vi "AVI Codec Comparison.vi"() -> ()   [LabVIEW 2014]
doc: "This example creates a new AVI for each compression filter installed on your computer and compares the size of the AVI file, the average write time, and the quality of the compressed AVI.\n\nThis example might take a few seconds to create all the AVIs required for analysis. The VI saves the AVIs in the temporary directory, which you set by selecting Tools>>Options, then selecting Paths from the top drop-down listbox."
uses:
  <vilib>/Analysis/baseanly.llb/Mean (DBL).vi
  <vilib>/vision/NI_Vision_Development_Module.lvlib
  <vilib>/Analysis/NI_AALBase.lvlib
panel:
  out "Results":i32(listbox)=-1
  out "Progress Bar":i32(slide) max=11 scale=0.0..11.0
  # "Overview: Demonstrates how to use the IMAQ AVI functions to compare the available codecs on the system and evaluate the codecs based on the resulting AVI size, write speed, and quality.\nRequirements: Vision Development Software.\nInstructions: Run the VI."
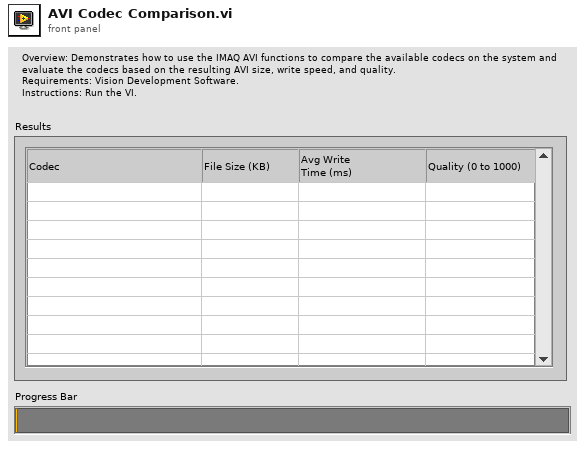
[diagram p1: front panel]
types:
  T1 = typedef "Image Type" = u32
  T2 = typedef "IMAQ Image.ctl" = refnum<image>
  T3 = typedef "IMAQ AVI2 Refnum.ctl" = refnum<k20>
  T4 = cluster{"histogram":u32[], "Minimal Value":sgl, "Maximal Value":sgl, "Starting Value":sgl, "Interval Width":sgl, "Mean Value":sgl, "Standard  Variation":sgl, "Area (pixels)":i32}
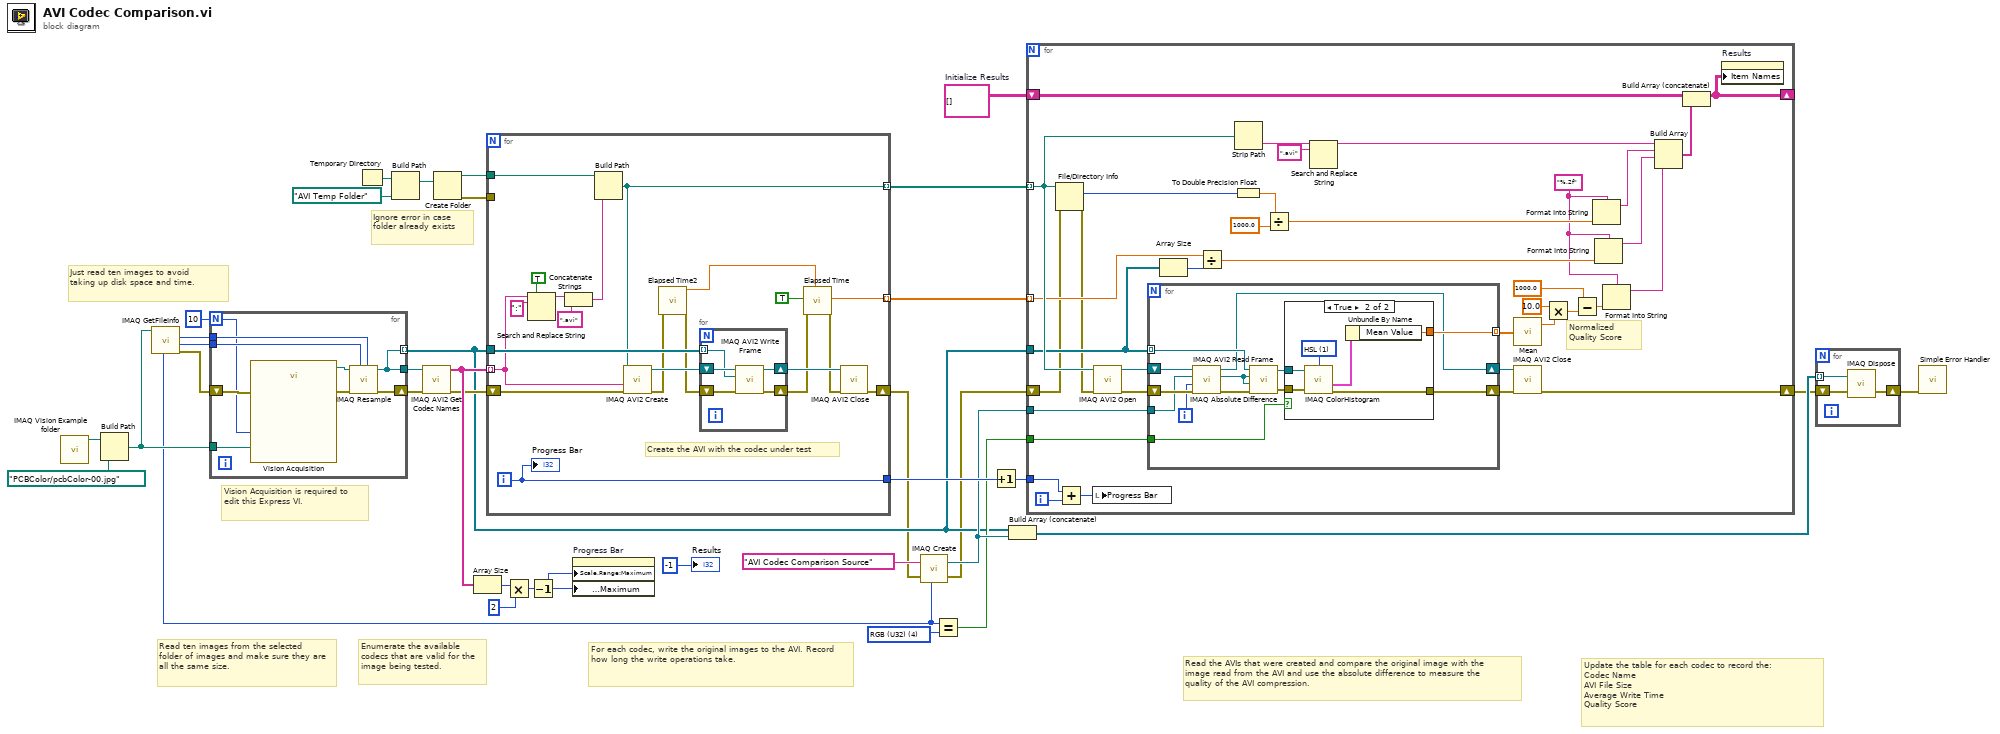
[diagram p0: block diagram]
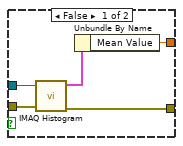
[diagram p2: hidden frame]
diagram:
  w18 = T1 4 items=["Grayscale (U8)", "Grayscale (I16)", "Grayscale (SGL)", "Complex (CSG)", "RGB (U32)", "HSL (U32)", "RGB (U64)", "Grayscale (U16)"] ("Image Type")
  w11 = string[][] []  # Initialize Results
  # "Ignore error in case folder already exists"
  # "Vision Acquisition is required to edit this Express VI."
  # "Update the table for each codec to record the:\nCodec Name\nAVI File Size\nAverage Write Time\nQuality Score"
  # "Read the AVIs that were created and compare the original image with the image read from the AVI and use the absolute difference to measure the quality of the AVI compression."
  # "For each codec, write the original images to the AVI. Record how long the write operations take."
  # "Enumerate the available codecs that are valid for the image being tested."
  # "Read ten images from the selected folder of images and make sure they are all the same size."
  # "Just read ten images to avoid taking up disk space and time."
  n1 = call "IMAQ Vision Example folder.vi"() -> ("Example Image Path"=w32:path)  [unwired: 11 in]
  n2 = Build Path(base path=w32, name or relative path=path "PCBColor/pcbColor-00.jpg") -> (appended path=w29:path)
  n3 = call "IMAQ GetFileInfo"("File Path"=w29) -> ("error out"=w28:errorcluster, "Y Resolution"=w26:i32, "X Resolution"=w27:i32, "Image Type"=w19:T1)  [unwired: 4 in, 3 out]
  n4 = for {
    N: 10 -> [w40]
    tunnel: w29 -> [w41]
    tunnel: [w45] -> w6 mode=indexing
    shift-right: [w46] -> w2
    shift-left: w28 -> [w42]
    tunnel: [w45] -> w25
    tunnel: w27 -> [w44]
    tunnel: w26 -> [w43]
    n5 = call "Vision Acquisition"("Image Path"=w41, "Number of Images"=w40, "error in"=w42) -> ("Image Out"=w38:T2, "error out"=w39:errorcluster)  [unwired: 21 in, 2 out]
    n6 = call "IMAQ Resample"("X Resolution"=w44, "Y Resolution"=w43, "error in (no error)"=w39, "Image Src"=w38) -> ("error out"=w46:errorcluster, "Image Dst Out"=w45:T2)  [unwired: 6 in]
  }
  n7 = Temporary Directory() -> (w3:path)
  n8 = Build Path(base path=w3, name or relative path=path "AVI Temp Folder") -> (appended path=w36:path)
  n9 = call "IMAQ AVI2 Get Codec Names"("error in (no error)"=w2, "Image"=w25) -> ("error out"=w24:errorcluster, "Codec Names"=w33:string[])  [unwired: 1 in, 7 out]
  n10 = Create Folder(path (use dialog)=w36) -> (created path=w35:path, error out=w1:errorcluster)  [unwired: 1 in, 2 out]
  n11 = Array Size(array=w33) -> (size(s)=w23:i32)
  n12 = for "This loop creates a new AVI for each compressor installed on your machine.\nThe new AVI copies images from an original uncompressed AVI.  While the frames are being copied,\nthe average write time is recorded.  When the AVI is finished writing, the file size is recorded and it is compared\nwith the original AVI to see how similar it is using a simple subtraction. \nThe average write time, file size, and quality are recorded in the Results table." {
    tunnel: w35 -> [w67]
    tunnel: w33 -> [w60] mode=indexing
    tunnel: w6 -> [w62]
    tunnel: [w52] -> w17 mode=indexing
    tunnel: [w50] -> w16 mode=indexing
    shift-right: [w48] -> w5
    shift-left: w24 -> [w65]
    tunnel: [w49] -> w10
    tunnel: w1 -> [_]
    i -> [w49]
    # "Create the AVI with the codec under test"
    n13 = Search and Replace String(replace all?=TRUE ("replace all? (F)"), input string=w60, search string=":" ("regular expression (\"\")")) -> (result string=w58:string)  [unwired: 5 in, 3 out]
    n14 = Concatenate Strings(w58, ".avi" ("Substring")) -> (w66:string)
    n15 = Build Path(base path=w67, name or relative path=w66) -> (appended path=w52:path)
    n16 = call "IMAQ AVI2 Create"("error in (no error)"=w65, "Codec"=w60, "AVI Path"=w52) -> ("error out"=w56:errorcluster, "AVI Refnum"=w63:T3)  [unwired: 2 in, 5 out]
    n17 = call "Elapsed Time2"("error in (no error)"=w56) -> ("Present (s)"=w51:dbl, "error out"=w53:errorcluster)  [unwired: 11 in, 6 out]
    n18 = for {
      tunnel: w62 -> [w70] mode=indexing
      shift-right: [w69] -> w57
      shift-left: w63 -> [w71]
      shift-right: [w68] -> w55
      shift-left: w53 -> [w72]
      n19 = call "IMAQ AVI2 Write Frame"("error in (no error)"=w72, "Image"=w70, "AVI Refnum"=w71) -> ("error out"=w68:errorcluster, "AVI Refnum (duplicate)"=w69:T3)  [unwired: 7 out]
    }
    n20 = call "Elapsed Time"("Reset"=TRUE, "error in (no error)"=w55, "Set Start Time (s)"=w51) -> ("Elapsed Time (s)"=w50:dbl, "error out"=w54:errorcluster)  [unwired: 9 in, 6 out]
    n21 = call "IMAQ AVI2 Close"("error in (no error)"=w54, "AVI Refnum"=w57) -> ("error out"=w48:errorcluster)  [unwired: 9 out]
    "Progress Bar" <- w49
  }
  n22 = Multiply(x=w23, y=2) -> (x*y=w21:i32)
  n23 = Decrement(x=w21) -> (x-1=w34:i32)
  n24 = property on="Progress Bar" class="Slide (strict)"("Scale.Range:Maximum"=w34, "Data Entry Limits:Maximum"=w34) -> ()  [unwired: 2 in, 2 out]
  n25 = call "IMAQ Create"("Image Name"="AVI Codec Comparison Source", "Image Type"=w19, "error in (no error)"=w5) -> ("New Image"=w8:T2, "error out"=w4:errorcluster)  [unwired: 1 in, 1 out]
  n26 = Equal?(x=w19, y=w18) -> (x = y?=w7:bool)
  n27 = Increment(x=w10) -> (x+1=w9:i32)
  n28 = Build Array (concatenate)(w6, w8) -> (w15:T2[])
  n29 = for {
    tunnel: w17 -> [w108] mode=indexing
    tunnel: w16 -> [w98] mode=indexing
    shift-right: [w78] -> w13
    shift-left: w4 -> [w74]
    tunnel: w6 -> [w97]
    shift-right: [w84] -> _
    shift-left: w11 -> [w86]
    tunnel: w9 -> [w77]
    tunnel: w8 -> [w76]
    tunnel: w7 -> [w75]
    i -> [w83]
    w88 = "%.2f" ("format string")
    # "Normalized Quality Score"
    n30 = File/Directory Info(path=w108, error in=w74) -> (size=w105:i64, error out=w73:errorcluster)  [unwired: 5 out]
    n31 = Add(x=w77, y=w83) -> (x+y=w82:i32)
    n32 = local write "Progress Bar"(w82) -> ()
    n33 = call "IMAQ AVI2 Open"("error in (no error)"=w73, "AVI File Path"=w108) -> ("error out"=w109:errorcluster, "AVI Refnum"=w80:T3)  [unwired: 8 in]
    n34 = for {
      tunnel: w97 -> [w118] mode=indexing
      tunnel: [w115] -> w100 mode=indexing
      shift-right: [w114] -> w81
      shift-left: w109 -> [w121]
      shift-right: [w112] -> w79
      shift-left: w80 -> [w122]
      tunnel: w76 -> [w111]
      tunnel: w75 -> [w110]
      i -> [w120]
      n35 = call "IMAQ AVI2 Read Frame"("error in (no error)"=w121, "Frame Number"=w120, "Image"=w111, "AVI Refnum"=w122) -> ("error out"=w119:errorcluster, "Image Out"=w113:T2, "AVI Refnum (duplicate)"=w112:T3)  [unwired: 5 in]
      n36 = call "IMAQ Absolute Difference"("Image Src A"=w118, "Image Dst"=w113, "Image Src B"=w113, "error in (no error)"=w119) -> ("Image Dst Out"=w116:T2, "error out"=w117:errorcluster)  [unwired: 3 in]
      n37 = case shown="True" w110 {
        tunnel: w117 -> [w126 w132]
        tunnel: w116 -> [w127 w133]
        tunnel: [w124 w129] -> w115
        tunnel: [w123 w128] -> w114
        frame False {
          n38 = call "IMAQ Histogram"("error in (no error)"=w126, "Image"=w127) -> ("error out"=w123:errorcluster, "Histogram Report"=w125:T4)  [unwired: 8 in]
          n39 = Unbundle By Name(w125) -> ("Mean Value"=w124:sgl)
        }
        frame True {
          w131 = u16 1 items=["RGB", "HSL", "HSV", "HSI", "CIE L*a*b*", "CIE XYZ"] ("Color Mode")
          n40 = call "IMAQ ColorHistogram"("Color Mode"=w131, "Image Src"=w133, "error in (no error)"=w132) -> ("Blue or Luma or Val or Inten or Z or b* Histogram Report"=w130:T4, "error out"=w128:errorcluster)  [unwired: 3 in, 2 out]
          n41 = Unbundle By Name(w130) -> ("Mean Value"=w129:sgl)
        }
      }
    }
    n42 = Array Size(array=w97) -> (size(s)=w96:i32)
    n43 = Divide(x=w98, y=w96) -> (x/y=w95:dbl)
    n44 = Strip Path(path=w108) -> (name=w107:string)  [unwired: 1 out]
    n45 = To Double Precision Float(number=w105) -> (double precision float=w103:dbl)
    n46 = Divide(x=w103, y=1000.0) -> (x/y=w101:dbl)
    n47 = Search and Replace String(input string=w107, search string=".avi") -> (result string=w102:string)  [unwired: 6 in, 3 out]
    n48 = call-poly <vilib>:"Mean.vi"("X"=w100) -> ("mean"=w93:dbl)  [unwired: 1 out]
    n49 = call "IMAQ AVI2 Close"("error in (no error)"=w81, "AVI Refnum"=w79) -> ("error out"=w78:errorcluster)  [unwired: 9 out]
    n50 = Multiply(x=10.0, y=w93) -> (x*y=w90:dbl)
    n51 = Subtract(x=1000.0, y=w90) -> (x-y=w89:dbl)
    n52 = Format Into String(format string=w88, w101) -> (resulting string=w99:string)  [unwired: 2 in, 1 out]
    n53 = Format Into String(format string=w88, w95) -> (resulting string=w94:string)  [unwired: 2 in, 1 out]
    n54 = Format Into String(format string=w88, w89) -> (resulting string=w87:string)  [unwired: 2 in, 1 out]
    n55 = Build Array(w102, w99, w94, w87) -> (w85:string[])
    n56 = Build Array (concatenate)(w86, w85) -> (w84:string[][])
    n57 = property on="Results" class="MCListbox (strict)"("Item Names"=w84) -> ()  [unwired: 2 in, 2 out]
  }
  n58 = for {
    shift-right: [w135] -> w14
    shift-left: w13 -> [w136]
    tunnel: w15 -> [w134] mode=indexing
    n59 = call "IMAQ Dispose"("Image"=w134, "error in (no error)"=w136) -> ("error out"=w135:errorcluster)  [unwired: 1 in, 3 out]
  }
  n60 = call <vilib>:"Simple Error Handler.vi"("error in (no error)"=w14) -> ()  [unwired: 1 in, 8 out]
  "Results" <- -1 ("Results")
